vi "String.Parse Substring with Start and End Delimiter.vi"(9 "Delimiter2":string, 10 "Delimiter1":string, 11 "String In":string) -> (1 "Found":bool, 3 "String Out":string)   [LabVIEW 2024]
uses:
  <vilib>/Utility/error.llb/Trim Whitespace One-Sided.vi
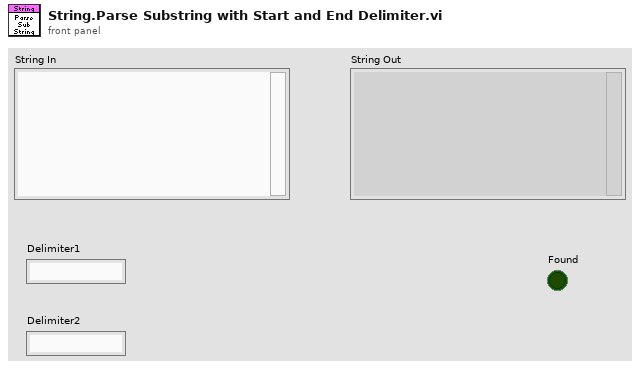
[diagram p1: front panel]
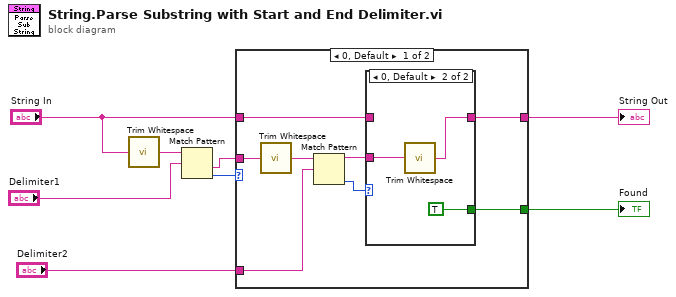
[diagram p0: block diagram]
diagram:
  n1 = call <vilib>:"Trim Whitespace.vi"("string"="String In") -> ("trimmed string"=w8:string)  [unwired: 1 in]
  n2 = Match Pattern(string=w8, regular expression="Delimiter1") -> (after substring=w5:string, offset past match=w6:i32)  [unwired: 1 in, 2 out]
  n3 = case shown="0, Default" w6 {
    tunnel: w5 -> [w15 _]
    tunnel: "Delimiter2" -> [w14 _]
    tunnel: [w12 w21] -> w2
    tunnel: "String In" -> [w11 w21]
    tunnel: [w10 _] -> w1
    frame 0, Default {
      n4 = call <vilib>:"Trim Whitespace.vi"("string"=w15) -> ("trimmed string"=w16:string)  [unwired: 1 in]
      n5 = Match Pattern(string=w16, regular expression=w14) -> (before substring=w9:string, offset past match=w13:i32)  [unwired: 1 in, 2 out]
      n6 = case shown="0, Default" w13 {
        tunnel: w9 -> [_ w20]
        tunnel: [w17 w19] -> w12
        tunnel: w11 -> [w17 _]
        tunnel: [_ TRUE] -> w10
        frame -1 {
        }
        frame 0, Default {
          n7 = call <vilib>:"Trim Whitespace.vi"("string"=w20) -> ("trimmed string"=w19:string)  [unwired: 1 in]
        }
      }
    }
    frame -1 {
    }
  }
  "String Out" <- w2
  "Found" <- w1
